vi "Event Info to Dqmh Event.vi"(8 "error in":errorcluster, 11 "Event Info":T1[](array[typedef])) -> (0 "error out":errorcluster, 3 "Dqmh Event":refnum<class "Dqmh Event.lvclass">[](array[class]))   [LabVIEW 2021, in "TAF Proj Document Type.lvlib" / "Project Parser.lvlib"]
uses:
  <vilib>/Wovalab/AntiDoc/Document Type/Add-ons/LabVIEW TAF Project/Project Parser/Project Parser.lvlib
  <vilib>/Wovalab/AntiDoc/Document Type/Add-ons/LabVIEW TAF Project/Project Parser/Dqmh Event Info--cluster.ctl
  <vilib>/Wovalab/AntiDoc/Document Type/Add-ons/LabVIEW TAF Project/Project Parser/Dqmh Event Type--enum.ctl
  <vilib>/Wovalab/AntiDoc/Document Type/Add-ons/LabVIEW TAF Project/Project Parser/Dqmh Event Links--cluster.ctl
  <vilib>/picture/picture.llb/imagedata.ctl
  <vilib>/Wovalab/AntiDoc/Document Type/Add-ons/LabVIEW TAF Project/Dqmh Event/Dqmh Event.lvclass
  C:/Program Files (x86)/National Instruments/LabVIEW 2021/vi.lib/Wovalab/AntiDoc/Document Type/Add-ons/LabVIEW TAF Project/Vi/Vi.lvclass
  <vilib>/Wovalab/AntiDoc/Document Type/Add-ons/LabVIEW TAF Project/Vi/Vi Info--cluster.ctl
  <vilib>/Wovalab/AntiDoc/Document Type/Add-ons/LabVIEW TAF Project/Dqmh Event/Dqmh Event.lvclass/Dqmh Event.ctl
  <vilib>/Wovalab/AntiDoc/Document Type/Add-ons/LabVIEW TAF Project/Dqmh Event/Write Event Type.vi
  <vilib>/Wovalab/AntiDoc/Document Type/Add-ons/LabVIEW TAF Project/Vi/Vi.lvclass
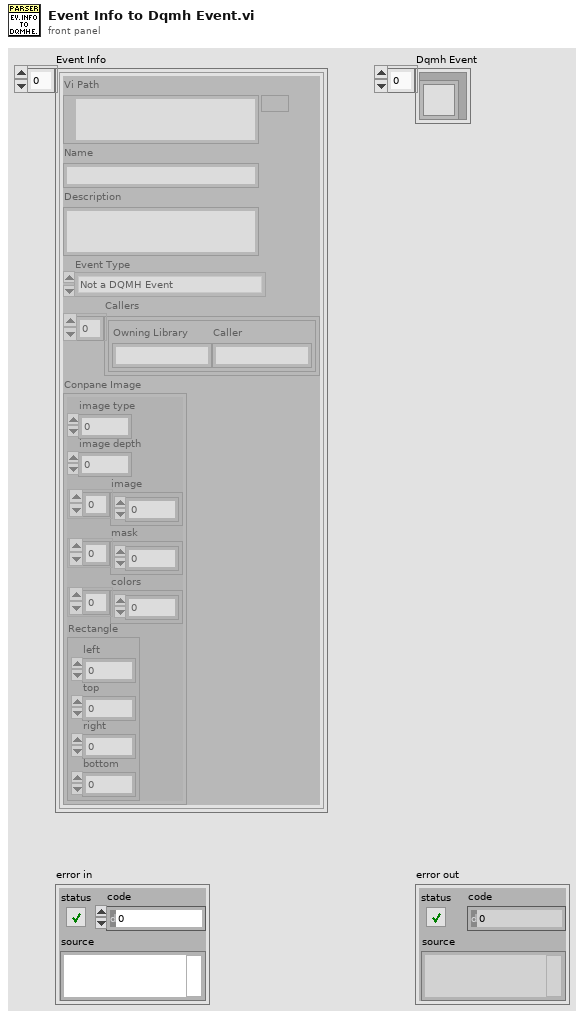
[diagram p1: front panel]
types:
  T1 = typedef "TAF Proj Document Type.lvlib/Project Parser.lvlib/Dqmh Event Info--cluster.ctl" = cluster{"Vi Path":path, "Name":string, "Description":string, "Event Type":T2, "Callers":T3[], "Conpane Image":T4}
  T2 = typedef "TAF Proj Document Type.lvlib/Project Parser.lvlib/Dqmh Event Type--enum.ctl" = enum16{"Not a DQMH Event", "Request", "Request And Wait For Reply", "Broadcast"}
  T3 = typedef "TAF Proj Document Type.lvlib/Project Parser.lvlib/Dqmh Event Links--cluster.ctl" = cluster{"Owning Library":string, "Caller":string}
  T4 = typedef "imagedata.ctl" = cluster{"image type":i32, "image depth":i32, "image":u8[], "mask":u8[], "colors":u32[], "Rectangle":cluster{"left":i16, "top":i16, "right":i16, "bottom":i16}}
  T5 = typedef "TAF Proj Document Type.lvlib/Vi.lvclass/Vi Info--cluster.ctl" = cluster{"Name":string, "Description":string, "Is Reentrant":bool, "Reentrancy Type":enum16{"Share clones between instances", "Preallocate clone for each instance"}, "Inline SubVI":bool, "Access Scope":enum32{"invalid scope", "public", "private", "protected", "community"}, "Conpane Image":T4}
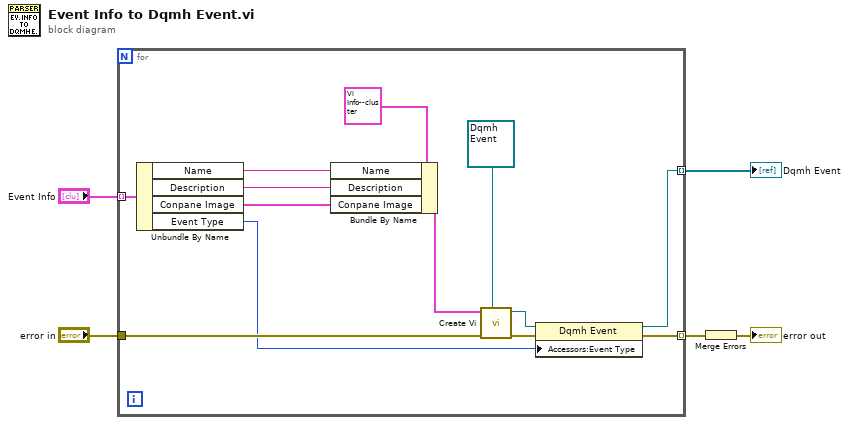
[diagram p0: block diagram]
diagram:
  n1 = for {
    tunnel: "Event Info" -> [w15] mode=indexing
    tunnel: [w14] -> w2 mode=indexing
    tunnel: "error in" -> [w17]
    tunnel: [w16] -> w1 mode=indexing
    n2 = Unbundle By Name(w15) -> ("Name"=w8:string, "Description"=w7:string, "Conpane Image"=w6:T4, "Event Type"=w13:T2)
    n3 = Bundle By Name(cluster=T5 {"Name"="", "Description"="", "Is Reentrant"=FALSE, "Reentrancy Type"=enum."Share clones between instances", "Inline SubVI"=FALSE, "Access Scope"=enum."invalid scope", "Conpane Image"={"image type"=0, "image depth"=0, "image"=[], "mask"=[], "colors"=[], "Rectangle"={"left"=0, "top"=0, "right"=0, "bottom"=0}}} ("Vi Info"), "Name"=w8, "Description"=w7, "Conpane Image"=w6) -> (w9:T5)
    n4 = call <vilib>:"Create Vi.vi"("Vi Type"=refnum<class "Dqmh Event.lvclass"> refnum ("Dqmh Event.lvclass"), "error in"=w17, "Vi Info"=w9) -> ("error out"=w18:errorcluster, "Vi out"=w11:refnum<class "Dqmh Event.lvclass">)  [unwired: 7 in]
    n5 = property class="Dqmh Event"(reference=w11, error in=w18, "Accessors:Event Type"=w13) -> (reference out=w14:refnum<class "Dqmh Event.lvclass">, error out=w16:errorcluster)
  }
  "Dqmh Event" <- w2
  n6 = Merge Errors(w1) -> (→"error out":errorcluster)
